vi "AcqLoop.vi"(8 "error in (no error)":errorcluster, 11 "DemoStage in":refnum<class "DemoStage.lvclass">) -> (0 "error out":errorcluster, 3 "DemoStage out":refnum<class "DemoStage.lvclass">)   [LabVIEW 2020, in "DemoStage.lvlib" / "DemoStage.lvclass"]
uses:
  DemoStage.lvclass
  C:/Program Files/National Instruments/LabVIEW 2020/vi.lib/ActorFramework/Actor/Actor.lvclass
  Hardware Abstraction Layer/Component/Device/Device/DeviceStatus.ctl
  <vilib>/ActorFramework/Message Enqueuer/Message Priority.ctl
  <vilib>/ActorFramework/Actor/Actor.lvclass/Actor.ctl
  <vilib>/ActorFramework/Message Enqueuer/Message Enqueuer.lvclass/Message Enqueuer.ctl
  <vilib>/ActorFramework/Message Enqueuer/Init from Existing Queue.vi
  <vilib>/ActorFramework/Message Enqueuer/Enqueue.vi
  Hardware Abstraction Layer/Component/Device/Device Messages/AcqLoop Msg/AcqLoop Msg.lvclass
  C:/Program Files/National Instruments/LabVIEW 2020/vi.lib/ActorFramework/Message/Message.lvclass
  <vilib>/ActorFramework/Message Priority Queue/Priority Enqueue.vi
  Hardware Abstraction Layer/Component/Stage/Stage/Stage.lvclass
  <vilib>/ActorFramework/Message Enqueuer/Message Enqueuer.lvclass
  Hardware Abstraction Layer/Component/Device/Device/Device.lvlib
  <vilib>/ActorFramework/Actor/Actor.lvclass
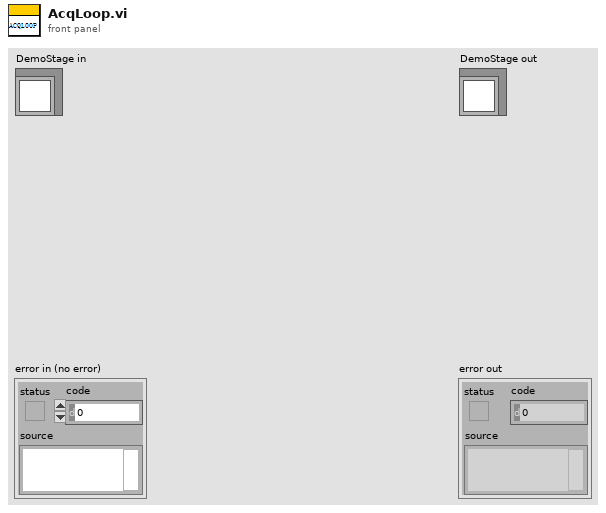
[diagram p1: front panel]
types:
  T1 = typedef "Actor Framework.lvlib/Message Enqueuer.lvclass/Message Priority.ctl" = enum16{"Low", "Normal", "High"}
  T2 = typedef "DataListener.lvclass/DataExchange.ctl" = cluster{"Source":string, "Destination":string, "Description":string, "value":variant}
  T3 = typedef "Device.lvlib/DeviceStatus.ctl" = i32
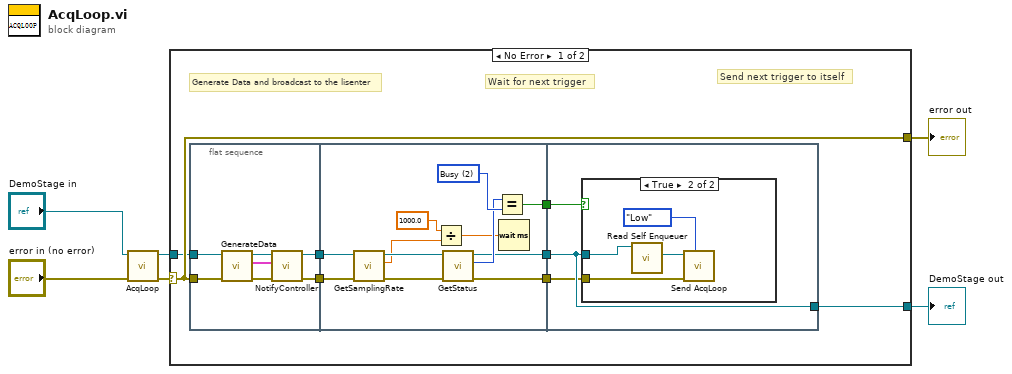
[diagram p0: block diagram]
diagram:
  n1 = call-parent "AcqLoop.vi"("error in (no error)"="error in (no error)", "Device in"="DemoStage in") -> ("error out"=w3:errorcluster, "Device out"=w4:refnum<class "DemoStage.lvclass">)  [unwired: 8 in]
  n2 = case shown="No Error" w3 {
    selector: w3 -> [w9 w42]
    tunnel: [w9 w42] -> w1
    tunnel: [w7 w41] -> w2
    tunnel: w4 -> [w8 w41]
    frame No Error {
      # "Send next trigger to itself"
      # "Wait for next trigger"
      # "Generate Data and broadcast to the lisenter"
      n3 = flat-sequence {
        tunnel: w8 -> [w21]
        tunnel: w9 -> [w19]
        tunnel: [w18] -> w14
        tunnel: [w15] -> w13
        tunnel: w14 -> [w26]
        tunnel: [w28] -> w12
        tunnel: w13 -> [w31]
        tunnel: [w33] -> w11
        tunnel: [w30] -> w10
        tunnel: [w35] -> w7
        tunnel: w12 -> [w35]
        tunnel: w11 -> [w36]
        tunnel: w10 -> [w34]
        frame #0 {
          n4 = call-dynamic "GenerateData.vi"("error in (no error)"=w19, "DemoStage in"=w21) -> ("error out"=w16:errorcluster, "DataExchange"=w17:T2, "DemoStage out"=w20:refnum<class "DemoStage.lvclass">)  [unwired: 7 in]
          n5 = call-dynamic "NotifyController.vi"("error in (no error)"=w16, "DataExchange"=w17, "Device in"=w20) -> ("error out"=w15:errorcluster, "Device out"=w18:refnum<class "DemoStage.lvclass">)  [unwired: 7 in]
        }
        frame #1 {
          w32 = T3 2 items=["Offline", "Idle", "Busy"] ("y")
          n6 = call-dynamic "GetSamplingRate.vi"("error in (no error)"=w31, "Device in"=w26) -> ("error out"=w27:errorcluster, "SamplingRate"=w22:dbl, "Device out"=w25:refnum<class "DemoStage.lvclass">)  [unwired: 7 in]
          n7 = Divide(x=1000.0, y=w22) -> (x/y=w24:dbl)
          n8 = call-dynamic "GetStatus.vi"("error in (no error)"=w27, "Device in"=w25) -> ("error out"=w30:errorcluster, "Status"=w29:T3, "Device out"=w28:refnum<class "DemoStage.lvclass">)  [unwired: 7 in]
          n9 = Equal?(x=w29, y=w32) -> (x = y?=w33:bool)
          n10 = Wait (ms)(milliseconds to wait=w24) -> ()  [unwired: 1 out]
        }
        frame #2 {
          n11 = case shown="True" w36 {
            tunnel: w35 -> [_ w40]
            tunnel: w34 -> [_ w38]
            frame False {
            }
            frame True {
              n12 = call <vilib>:"Read Self Enqueuer.vi"("Actor"=w40) -> ("Self Enqueuer"=w39:refnum<class "Message Enqueuer.lvclass">)  [unwired: 10 in]
              n13 = call "Send AcqLoop.vi"("Message Priority (Normal)"=Message_Priority."Low", "error in (no error)"=w38, "Message Enqueuer"=w39) -> ()  [unwired: 7 in, 2 out]
            }
          }
        }
      }
    }
    frame Error {
    }
  }
  "error out" <- w1
  "DemoStage out" <- w2
